vi "Open Therm Connections.vi"(8 "error in (no error)":errorcluster, 9 "Attempt Connection? (T)":bool=TRUE, 10 "timeout (100ms)":i32=100, 11 "PSP Therm Channels in":refnum<k21>[](array[refnum])) -> (0 "error out":errorcluster, 1 "Successful Connections":string, 3 "Opened Variables out":refnum<k21>[](array[refnum]), 4 "Errors":errorcluster[](array[cluster]))   [LabVIEW 2018]
uses:
  <userlib>/_OpenG.lib/error/error.llb/Filter Error Codes (Array)__ogtk.vi
  RT - Instrument IO.lvlib
panel:
  out "Test Read":dbl
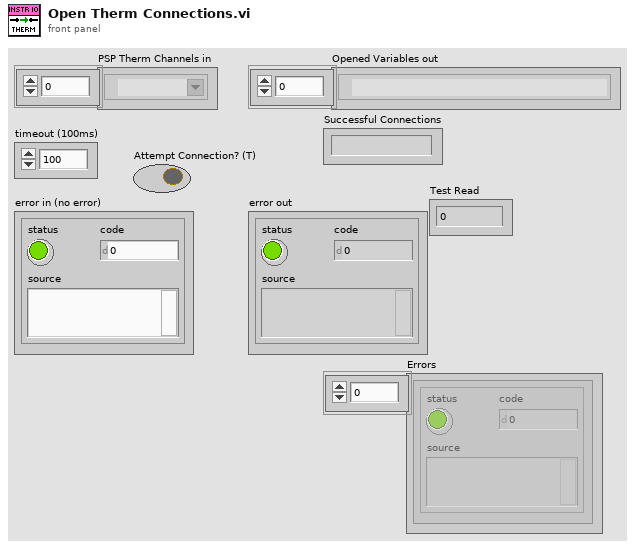
[diagram p1: front panel]
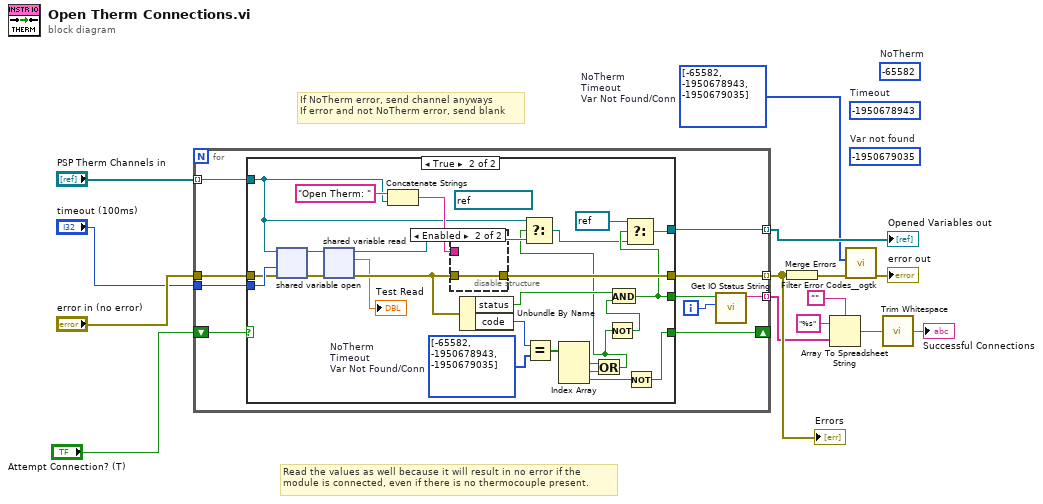
[diagram p0: block diagram]
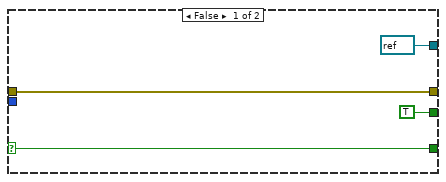
[diagram p2: hidden frame]
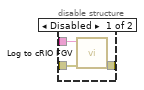
[diagram p3: hidden frame]
diagram:
  w1 = i32[] [-65582, -1950678943, -1950679035]  # NoTherm Timeout Var Not Found/Conn
  (unwired) -65582  # NoTherm
  (unwired) -1950678943  # Timeout
  (unwired) -1950679035  # Var not found
  # "If NoTherm error, send channel anyways\nIf error and not NoTherm error, send blank"
  # "Read the values as well because it will result in no error if the\nmodule is connected, even if there is no thermocouple present."
  n1 = for {
    tunnel: "PSP Therm Channels in" -> [w20] mode=indexing
    tunnel: [w21] -> w8 mode=indexing
    tunnel: [w24] -> w10 mode=indexing
    tunnel: "timeout (100ms)" -> [w23]
    tunnel: "error in (no error)" -> [w22]
    tunnel: [w17] -> w2 mode=indexing
    shift-right: [w18] -> _
    shift-left: "Attempt Connection? (T)" -> [w19]
    i -> [w15]
    n2 = case shown="True" w19 {
      selector: w19 -> [w26 _]
      tunnel: [refnum<k21> refnum ("shared variable refnum in") w41] -> w24
      tunnel: w23 -> [_ w52]
      tunnel: w22 -> [w27 w51]
      tunnel: [w27 w50] -> w21
      tunnel: w20 -> [_ w43]
      tunnel: [w26 w29] -> w18
      tunnel: [TRUE ("status") w42] -> w16
      frame False {
      }
      frame True {
        w37 = i32[] [-65582, -1950678943, -1950679035]  # NoTherm Timeout Var Not Found/Conn
        (unwired) refnum<k21> "NoTherm" ("t")
        n3 = shared-variable-open(w43, w51, w52) -> (w45:refnum<k21>, w53:errorcluster)  [unwired: 2 in]
        n4 = shared-variable-read(w45, w53) -> (w40:refnum<k21>, w47:errorcluster, →"Test Read":dbl)
        n5 = Concatenate Strings("Open Therm: " ("Line to Write(\"\")"), w43) -> (w48:string)
        n6 = disable-structure shown="Enabled" {
          disable-tunnel: [w56 w57] -> w50
          disable-tunnel: w48 -> [w55 _]
          disable-tunnel: w47 -> [w54 w57]
          frame Disabled {
            n7 = call "Log to cRIO FGV.vi"("error in"=w54, "Line to Write(\"\")"=w55) -> ("error out"=w56:errorcluster)  [unwired: 8 in, 1 out]
          }
          frame Enabled {
          }
        }
        n8 = Unbundle By Name(w47) -> ("status"=w44:bool, "code"=w36:i32)
        n9 = Equal?(x=w36, y=w37) -> (x = y?=w35:bool[])
        n10 = Index Array(array=w35) -> (element #1=w34:bool, element #2=w33:bool, element #3=w32:bool)  [unwired: 3 in]
        n11 = Or(x=w34, y=w33) -> (x .or. y?=w31:bool)
        n12 = Select(t=w43, s=w31, f=w40) -> (s? t:f=w38:refnum<k21>)
        n13 = Not(x=w31) -> (.not. x?=w30:bool)
        n14 = And(x=w44, y=w30) -> (x .and. y?=w42:bool)
        n15 = Select(t=refnum<k21> refnum, s=w42, f=w38) -> (s? t:f=w41:refnum<k21>)
        n16 = Not(x=w32) -> (.not. x?=w29:bool)
      }
    }
    n17 = call "Get IO Status String.vi"("Loop Index"=w15, "Error Status"=w16) -> ("Output String"=w17:string)  [unwired: 9 in]
  }
  "Opened Variables out" <- w10
  "Errors" <- w8
  n18 = Merge Errors(w8) -> (w9:errorcluster)
  n19 = Array To Spreadsheet String(delimiter (Tab)="", array=w2, 3:"%s" ("format string")) -> (spreadsheet string=w4:string)
  n20 = call-poly <userlib>:"Filter Error Codes__ogtk.vi"("Error In"=w9, "Error Codes to Filter"=w1) -> ("Error Out"=→"error out":errorcluster)  [unwired: 7 in, 2 out]
  n21 = call <vilib>:"Trim Whitespace.vi"("string"=w4) -> ("trimmed string"=→"Successful Connections":string)  [unwired: 1 in]
